vi "insert.vi"(8 "error in (no error)":errorcluster, 11 "DL090215DataCollection in":refnum<class "DataCollectionDL090215.lvclass">) -> (0 "error out":errorcluster, 3 "DL090215DataCollection out":refnum<class "DataCollectionDL090215.lvclass">)   [LabVIEW 2010, in "DataCollectionDL090215.lvclass"]
uses:
  DataCollectionDL090215.lvclass
  common/classes/Image/Image/Image.lvclass
  DataCollectionDL090215.lvclass/DataCollectionDL090215.ctl
  common/classes/ImageCollection/ImageCollection/ImageCollection.lvclass
  common/classes/ImageCollection/ImageCollection/add_mode_enum.ctl
  common/classes/GenericComponent/GenericComponent/class_data.vi
  common/classes/ErrorController/ErrorController/class_data.vi
  common/classes/ErrorController/ErrorController/ErrorController.lvclass
  common/classes/GenericComponent/GenericComponent/GenericComponent.lvclass
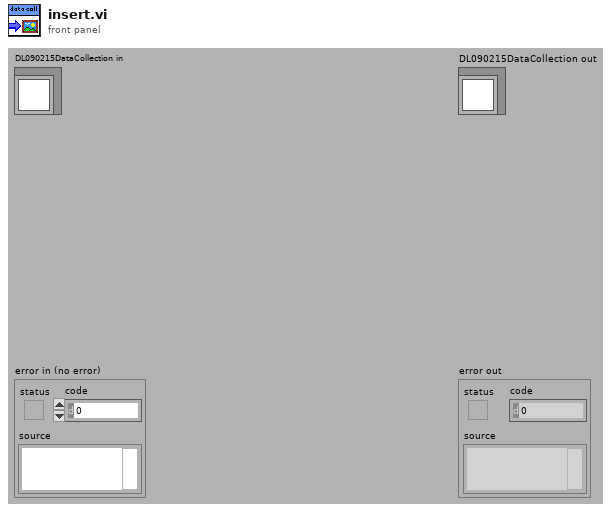
[diagram p1: front panel]
types:
  T1 = typedef "ImageCollection.lvclass/add_mode_enum.ctl" = enum16{"instance", "copy"}
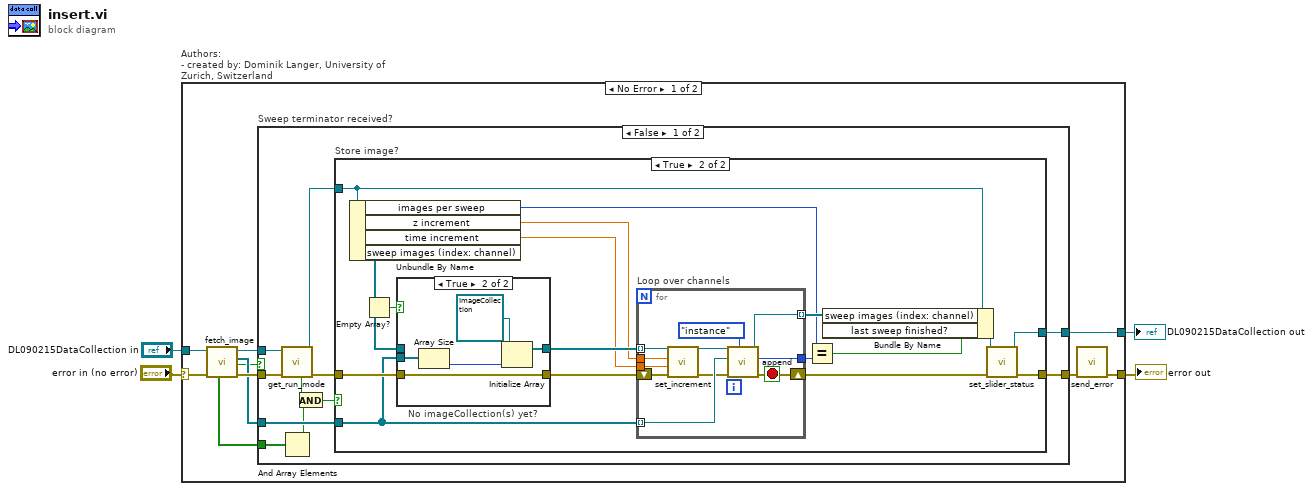
[diagram p0: block diagram]
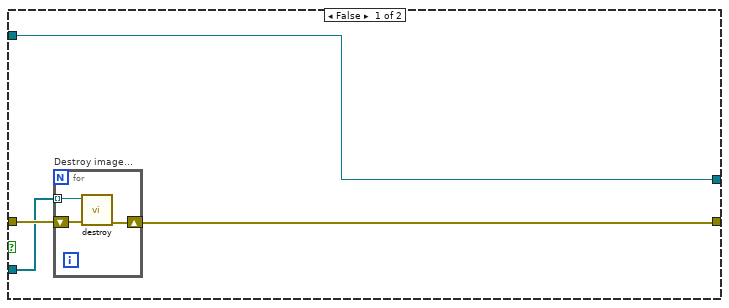
[diagram p2: hidden frame]
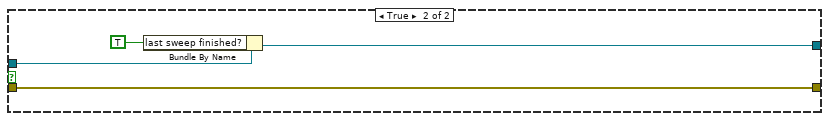
[diagram p4: hidden frame]
diagram:
  n1 = case "Authors: \n- created by: Dominik Langer, University of Zurich, Switzerland" shown="No Error" "error in (no error)" {
    selector: "error in (no error)" -> [w13 w73]
    tunnel: [w14 w73] -> w3
    tunnel: [w5 w72] -> w1
    tunnel: "DL090215DataCollection in" -> [w12 w72]
    frame No Error {
      n2 = call-dynamic "fetch_image.vi"("error in (no error)"=w13, "GenericToplevelComponent in"=w12) -> ("error out"=w11:errorcluster, "channels array empty?"=w7:bool, "image (channels)"=w9:refnum<class "Image.lvclass">[], "GenericToplevelComponent out"=w10:refnum<class "DataCollectionDL090215.lvclass">, "finished?"=w8:bool[])  [unwired: 4 in, 1 out]
      n3 = case "Sweep terminator received?" shown="False" w7 {
        tunnel: [w25 w68] -> w6
        tunnel: [w24 w71] -> w5
        tunnel: w10 -> [w16 w69]
        tunnel: w11 -> [w21 w68]
        tunnel: w9 -> [w23 _]
        tunnel: w8 -> [w22 _]
        frame False {
          n4 = call "get_run_mode.vi"("error in (no error)"=w21, "GenericPlugin in"=w16) -> ("error out"=w20:errorcluster, "GenericPlugin out"=w15:refnum<class "DataCollectionDL090215.lvclass">, "is NOT free run?"=w18:bool)  [unwired: 5 in, 2 out]
          n5 = And Array Elements(Boolean array=w22) -> (logical AND=w19:bool)
          n6 = And(x=w18, y=w19) -> (x .and. y?=w17:bool)
          n7 = case "Store image?" shown="True" w17 {
            tunnel: [w27 w49] -> w25
            tunnel: [w26 w48] -> w24
            tunnel: w15 -> [w26 w45]
            tunnel: w20 -> [w29 w41]
            tunnel: w23 -> [w28 w37]
            frame False {
              n8 = for "Destroy image..." {
                tunnel: w28 -> [w31] mode=indexing
                shift-right: [w30] -> w27
                shift-left: w29 -> [w32]
                n9 = call-dynamic "destroy.vi"("error in (no error)"=w32, "Image in"=w31) -> ("error out"=w30:errorcluster)  [unwired: 8 in, 1 out]
              }
            }
            frame True {
              n10 = Unbundle By Name(w45) -> ("images per sweep"=w33:i32, "z increment"=w35:dbl[unit], "time increment"=w34:dbl[unit], "sweep images (index: channel)"=w36:refnum<class "ImageCollection.lvclass">[])
              n11 = Empty Array?(array=w36) -> (empty?=w39:bool)
              n12 = case "No imageCollection(s) yet?" shown="True" w39 {
                tunnel: w41 -> [w51 w55]
                tunnel: [w51 w55] -> w40
                tunnel: [w50 w56] -> w38
                tunnel: w37 -> [_ w53]
                tunnel: w36 -> [w50 _]
                frame False {
                }
                frame True {
                  n13 = Array Size(array=w53) -> (size(s)=w52:i32)
                  n14 = Initialize Array(refnum<class "ImageCollection.lvclass"> refnum ("ImageCollection.lvclass"), w52) -> (w56:refnum<class "ImageCollection.lvclass">[])
                }
              }
              n15 = for "Loop over channels" {
                tunnel: w38 -> [w61] mode=indexing
                tunnel: w37 -> [w66] mode=indexing
                tunnel: [w67] -> w42 mode=indexing
                tunnel: [w64] -> w44
                shift-right: [w65] -> w46
                shift-left: w40 -> [w63]
                tunnel: w35 -> [w59]
                tunnel: w34 -> [w57]
                stop <- w65 stop-if-true
                n16 = call "set_increment.vi"("error in (no error)"=w63, "time increment"=w57, "z increment"=w59, "ImageCollection in"=w61) -> ("error out"=w62:errorcluster, "ImageCollection out"=w60:refnum<class "ImageCollection.lvclass">)  [unwired: 6 in]
                n17 = call-dynamic "append.vi"("add mode"=add_mode_enum."instance", "error in (no error)"=w62, "Image.lvclass"=w66, "ImageCollection in"=w60) -> ("error out"=w65:errorcluster, "new number of images"=w64:i32, "ImageCollection out"=w67:refnum<class "ImageCollection.lvclass">)  [unwired: 1 in, 4 out]
              }
              n18 = Equal?(x=w33, y=w44) -> (x = y?=w43:bool)
              n19 = Bundle By Name(cluster=w45, "sweep images (index: channel)"=w42, "last sweep finished?"=w43) -> (w47:refnum<class "DataCollectionDL090215.lvclass">)
              n20 = call-dynamic "set_slider_status.vi"("error in (no error)"=w46, "DL090215DataCollection in"=w47) -> ("error out"=w49:errorcluster, "DL090215DataCollection out"=w48:refnum<class "DataCollectionDL090215.lvclass">)  [unwired: 8 out]
            }
          }
        }
        frame True {
          n21 = Bundle By Name(cluster=w69, "last sweep finished?"=TRUE) -> (w71:refnum<class "DataCollectionDL090215.lvclass">)
        }
      }
      n22 = call "send_error.vi"("error in (no error)"=w6) -> ("error out"=w14:errorcluster)  [unwired: 10 in]
    }
    frame Error {
    }
  }
  "error out" <- w3
  "DL090215DataCollection out" <- w1
